vi "LS218_ENREGISTRER_CONFIG.vi"(4 "periode_acqui":i8, 5 "NOM MANIP":string, 6 "Type sondes 5-8":u16, 7 "Celsius":bool, 8 "entrée d'erreur (pas d'erreur)":errorcluster, 9 "Type sondes 1-4":u16, 10 "Voies de mesures":T1(array[cluster]), 11 "DOSSIER":path) -> (0 "sortie d'erreur":errorcluster)   [LabVIEW 2016]
uses:
  <vilib>/Utility/config.llb/Write Key (Boolean).vi
  <vilib>/Utility/config.llb/Write Key (Path).vi
  <vilib>/Utility/config.llb/Write Key (I32).vi
  <vilib>/Utility/config.llb/Write Key (String).vi
  <vilib>/Utility/config.llb/Write Key (U32).vi
  <vilib>/Utility/config.llb/NI_LVConfig.lvlib
panel:
  out "Tableau":string[](array[string])
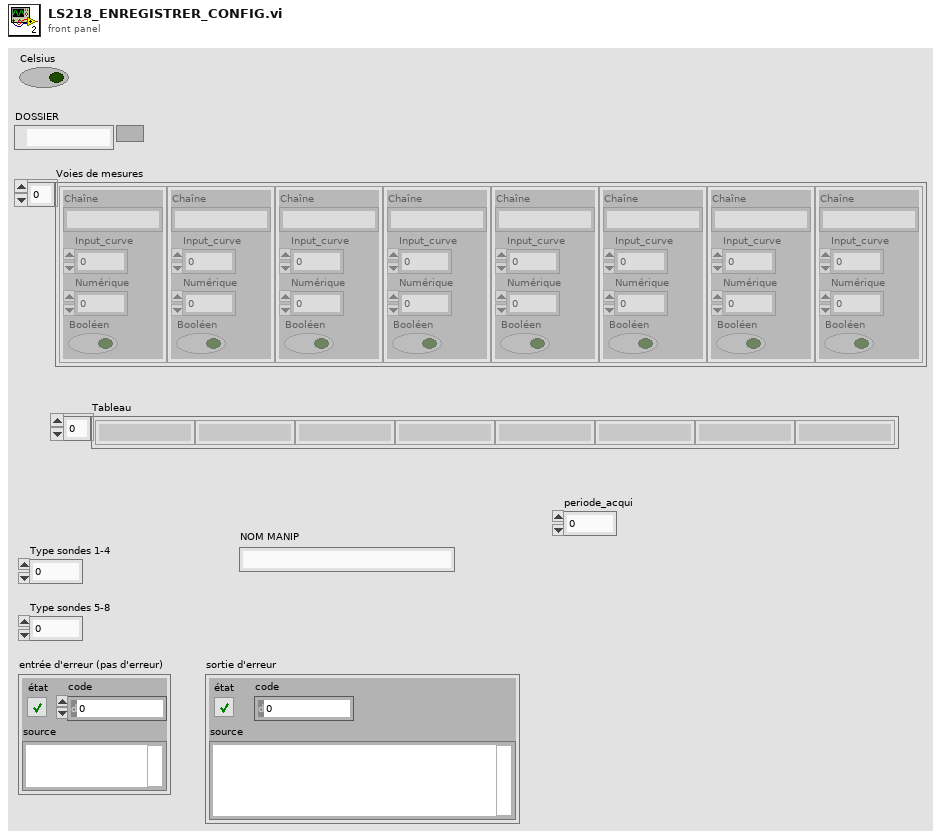
[diagram p1: front panel]
types:
  T1 = cluster{"Chaîne":string, "Input_curve":u16, "Numérique":dbl, "Booléen":bool}[]
  T2 = typedef "NI_LVConfig.lvlib/Config Data RefNum.ctl" = refnum<k1>
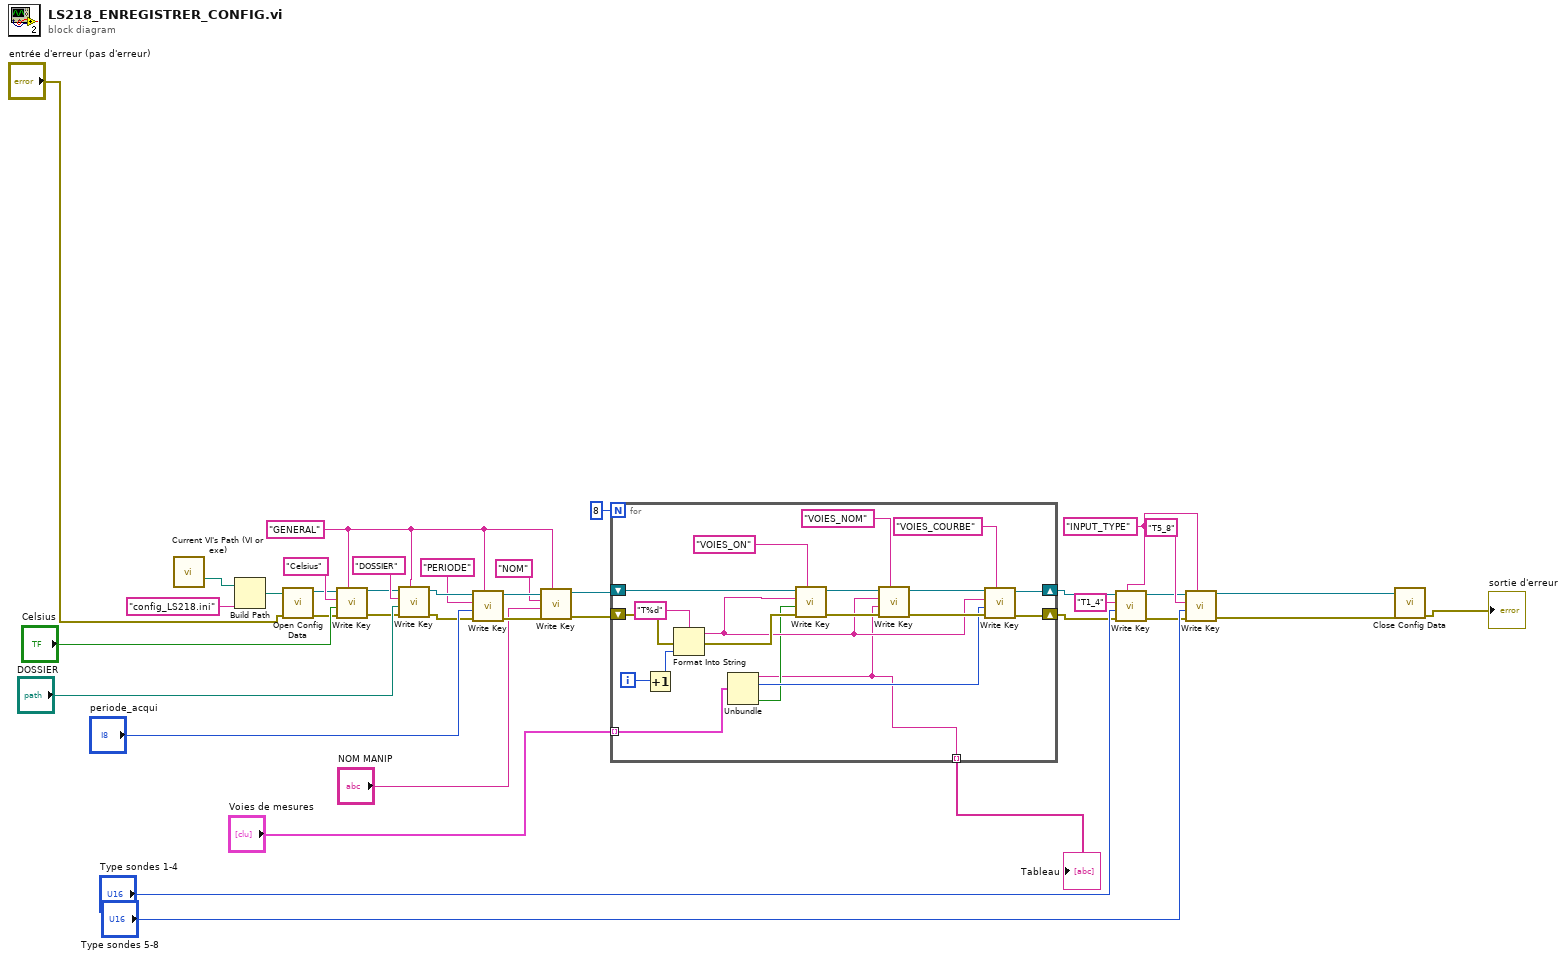
[diagram p0: block diagram]
diagram:
  w32 = "INPUT_TYPE" ("section")
  w3 = "GENERAL" ("section")
  n1 = call "Current VI's Path (VI or exe).vi"() -> ("VI or executable installation directory"=w13:path)  [unwired: 14 in, 1 out]
  n2 = Build Path(base path=w13, name or relative path="config_LS218.ini" ("nom ou chemin relatif")) -> (appended path=w15:path)
  n3 = call <vilib>:"Open Config Data.vi"("error in (no error)"="entrée d'erreur (pas d'erreur)", "configuration file path"=w15) -> ("error out"=w17:errorcluster, "refnum"=w16:T2)  [unwired: 7 in, 1 out]
  n4 = call-poly <vilib>:"Write Key.vi"("section"=w3, "error in (no error)"=w17, "value"="Celsius", "key"="Celsius", "refnum"=w16) -> ("error out"=w20:errorcluster, "refnum out"=w19:T2)  [unwired: 4 in, 1 out]
  n5 = call-poly <vilib>:"Write Key.vi"("section"=w3, "error in (no error)"=w20, "value"="DOSSIER", "key"="DOSSIER", "refnum"=w19) -> ("error out"=w9:errorcluster, "refnum out"=w10:T2)  [unwired: 4 in, 1 out]
  n6 = call-poly <vilib>:"Write Key.vi"("section"=w3, "error in (no error)"=w9, "value"="periode_acqui", "key"="PERIODE", "refnum"=w10) -> ("error out"=w7:errorcluster, "refnum out"=w5:T2)  [unwired: 4 in, 1 out]
  n7 = call-poly <vilib>:"Write Key.vi"("section"=w3, "error in (no error)"=w7, "value"="NOM MANIP", "key"="NOM", "refnum"=w5) -> ("error out"=w6:errorcluster, "refnum out"=w4:T2)  [unwired: 4 in, 1 out]
  n8 = for {
    N: 8 -> [_]
    shift-right: [w49] -> w29
    shift-left: w4 -> [w58]
    shift-right: [w50] -> w26
    shift-left: w6 -> [w55]
    tunnel: "Voies de mesures" -> [w48] mode=indexing
    tunnel: [w39] -> w12 mode=indexing
    i -> [w53]
    n9 = Increment(x=w53) -> (x+1=w52:i32)
    n10 = Format Into String(format string="T%d" ("key"), error in=w55, w52) -> (resulting string=w43:string, error out=w54:errorcluster)  [unwired: 1 in]
    n11 = Unbundle(w48) -> ("Chaîne"=w39:string, "Input_curve"=w41:u16, "Booléen"=w40:bool)  [unwired: 1 out]
    n12 = call-poly <vilib>:"Write Key.vi"("section"="VOIES_ON", "error in (no error)"=w54, "value"=w40, "key"=w43, "refnum"=w58) -> ("error out"=w47:errorcluster, "refnum out"=w45:T2)  [unwired: 4 in, 1 out]
    n13 = call-poly <vilib>:"Write Key.vi"("section"="VOIES_NOM", "error in (no error)"=w47, "value"=w39, "key"=w43, "refnum"=w45) -> ("error out"=w46:errorcluster, "refnum out"=w44:T2)  [unwired: 4 in, 1 out]
    n14 = call-poly <vilib>:"Write Key.vi"("section"="VOIES_COURBE", "error in (no error)"=w46, "value"=w41, "key"=w43, "refnum"=w44) -> ("error out"=w50:errorcluster, "refnum out"=w49:T2)  [unwired: 4 in, 1 out]
  }
  "Tableau" <- w12
  n15 = call-poly <vilib>:"Write Key.vi"("section"=w32, "error in (no error)"=w26, "value"="Type sondes 1-4", "key"="T1_4", "refnum"=w29) -> ("error out"=w27:errorcluster, "refnum out"=w30:T2)  [unwired: 4 in, 1 out]
  n16 = call-poly <vilib>:"Write Key.vi"("section"=w32, "error in (no error)"=w27, "value"="Type sondes 5-8", "key"="T5_8", "refnum"=w30) -> ("error out"=w28:errorcluster, "refnum out"=w31:T2)  [unwired: 4 in, 1 out]
  n17 = call <vilib>:"Close Config Data.vi"("error in (no error)"=w28, "refnum"=w31) -> ("error out"=→"sortie d'erreur":errorcluster)  [unwired: 8 in, 1 out]
